vi "FSK_SEND_TEST.vi"() -> ()   [LabVIEW 2015]
doc: "Continuously generates a communication signal that starts immediately. The device is not synchronized to external Reference Clocks or time bases."
uses:
  <vilib>/Utility/error.llb/DialogType.ctl
  <instrlib>/niUSRP/niUSRP Write Tx Data (CDB).vi
panel:
  out "数据源长度":dbl=1000.0
  in  "码元速率":dbl=10000.0
  in  "信号长度":dbl=50000.0
  out "实际发射帧数":dbl=50.0 format="%#_6f"
  in  "设定发射帧数":dbl=50.0
  in  "数据源文件":path=path "C:/Users/admin/Desktop/USRP0902/USRP/Fsk/SendBit.mat"
  out "波形图":dbl[](graph)
  out "实际发射增益":dbl=10.0 format="%#_6f"
  in  "设备IP":refnum<k15>="192.168.10.2"
  in  "天线选择":string="TX1"
  in  "stop":bool
  out "实际载波频率":dbl=1000000000.0 format="%#_6p"
  out "实际基带采样率":dbl=200000.0 format="%#_6p"
  in  "设定发射增益":dbl=10.0 format="%#_6f"
  in  "设定载波频率":dbl=1000000000.0 format="%#_6p"
  in  "设定基带采样率":dbl=200000.0 format="%#_6p"
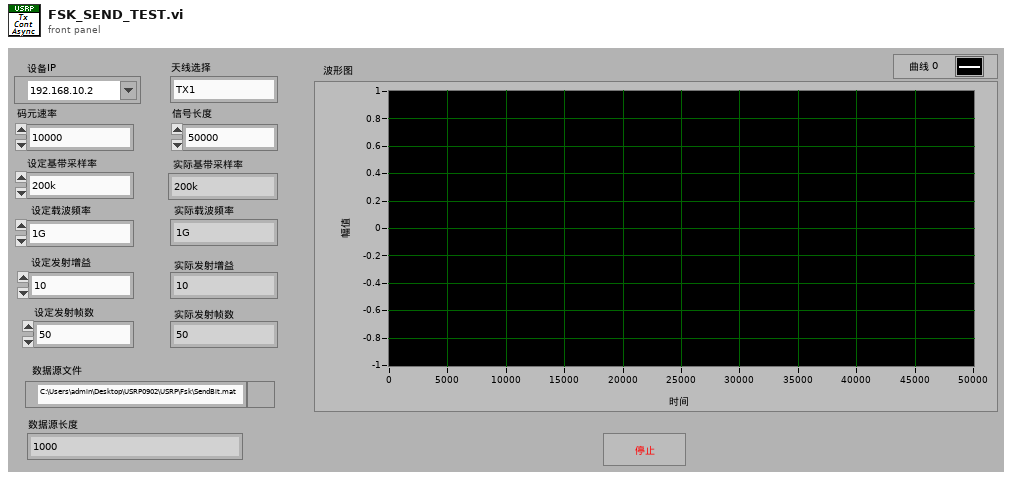
[diagram p1: front panel]
types:
  T1 = typedef "DialogType.ctl" = u16
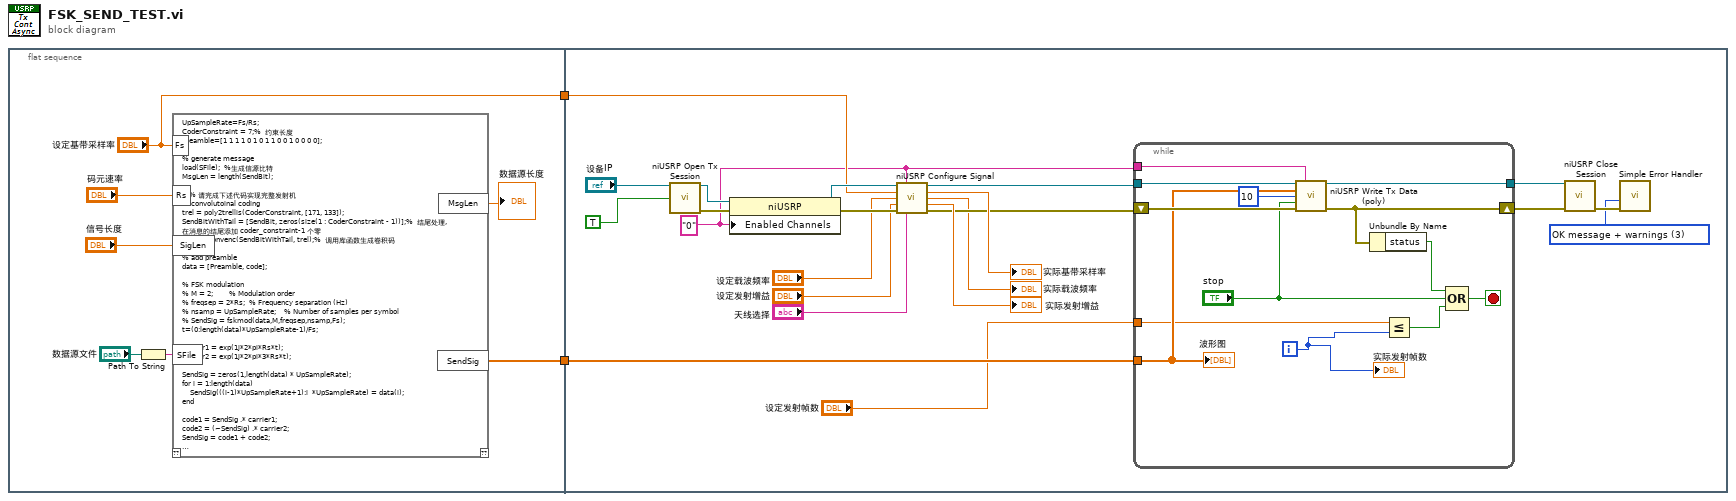
[diagram p0: block diagram]
diagram:
  n1 = flat-sequence {
    tunnel: ["设定基带采样率"] -> w2
    tunnel: [w6] -> w1
    tunnel: w2 -> [w13]
    tunnel: w1 -> [w12]
    frame #0 {
      n2 = Path To String(path="数据源文件") -> (string=w8:string)
      n3 = script code="UpSampleRate=Fs/Rs;\nCoderConstraint = 7;%  约束长度 \nPreamble=[1 1 1 1 0 1 0 1 1 0 0 1 0 0 0 0];\n\n% generate message\nload(SFile);  %生成信源比特\nMsgLen = length(SendBit);\n\n%% 请完成下述代码实现完整发射机\n% convolutoinal coding\ntrel = poly2trellis(CoderConstraint, [171, 133]);\nSendBitWithTail = [SendBit, zeros(size(1 : CoderConstraint - 1))];%  结尾处理, 在消息的结尾添加 coder_constraint-1 个零\ncode = convenc(SendBitWithTail, trel);%  调用库函数生成卷积码\n\n% add preamble \ndata = [Preamble, code];\n\n% FSK modulation\n% M = 2;        % Modulation order\n% freqsep = 2*Rs;  % Frequency separation (Hz)\n% nsamp = UpSampleRate;    % Number of samples per symbol\n% SendSig = fskmod(data,M,freqsep,nsamp,Fs);\nt=(0:length(data)*UpSampleRate-1)/Fs;\n\ncarrier1 = exp(1j*2*pi*Rs*t);\ncarrier2 = exp(1j*2*pi*3*Rs*t);\n\nSendSig = zeros(1,length(data) * UpSampleRate);\nfor i = 1:length(data)\n    SendSig(((i-1)*UpSampleRate+1):i  *UpSampleRate) = data(i);\nend\n\ncode1 = SendSig .* carrier1;\ncode2 = (~SendSig) .* carrier2;\nSendSig = code1 + code2;\n\n% 确保信号长度是SigLen\nif length(SendSig)>SigLen\n    SendSig = SendSig(1:SigLen);\nelseif length(SendSig)<SigLen\n    SendSig = [SendSig zeros(1,SigLen-length(SendSig))];\nend\nfigure;plot(SendBit);title('SendBit：数据源比特');\nfigure;plot(phasez(SendSig));title('phase(SendSig)：FSK发送信号相位');"("Fs"="设定基带采样率", "SFile"=w8, "Rs"="码元速率", "SigLen"="信号长度") -> ("SendSig"=w6:cdb[], "MsgLen"=→"数据源长度":dbl)  [unwired: 1 in, 1 out]
    }
    frame #1 {
      w11 = "0"
      w30 = T1 3 items=["no dialog", "OK message", "continue or stop message", "OK message + warnings", "continue/stop + warnings"] ("type of dialog (OK msg:1)")
      n4 = call <instrlib>:"niUSRP Open Tx Session.vi"("device names"="设备IP", "reset"=TRUE) -> ("session handle out"=w26:refnum<k15>, "error out"=w25:errorcluster)  [unwired: 12 in]
      n5 = property class="niUSRP"(reference=w26, error in=w25, "Enabled Channels"=w11) -> (reference out=w27:refnum<k15>, error out=w28:errorcluster)
      n6 = call <instrlib>:"niUSRP Configure Signal.vi"("session handle"=w27, "channel list"=w11, "IQ rate"=w13, "carrier frequency"="设定载波频率", "gain"="设定发射增益", "error in (no error)"=w28, "active antenna"="天线选择") -> ("session handle out"=w16:refnum<k15>, "coerced IQ rate"=→"实际基带采样率":dbl, "coerced carrier frequency"=→"实际载波频率":dbl, "coerced gain"=→"实际发射增益":dbl, "error out"=w17:errorcluster)  [unwired: 4 in]
      n7 = while {
        tunnel: w16 -> [w43]
        tunnel: [w41] -> w18
        shift-right: [w40] -> w19
        shift-left: w17 -> [w42]
        tunnel: w11 -> [w38]
        tunnel: w12 -> [w37]
        tunnel: "设定发射帧数" -> [w33]
        i -> [w32]
        stop <- w44 stop-if-true
        n8 = call-poly <instrlib>:"niUSRP Write Tx Data (poly).vi"("session handle"=w43, "channel list"=w38, "data"=w37, "timeout"=10, "end of data?"="stop", "error in (no error)"=w42) -> ("session handle out"=w41:refnum<k15>, "error out"=w40:errorcluster)  [unwired: 8 in]
        n9 = Unbundle By Name(w40) -> ("status"=w39:bool)
        n10 = Less Or Equal?(x=w33, y=w32) -> (x <= y?=w35:bool)
        n11 = Compound Arithmetic op=OR(w39, "stop", w35) -> (w44:bool)
        "波形图" <- w37
        "实际发射帧数" <- w32
      }
      n12 = call <instrlib>:"niUSRP Close Session.vi"("session handle"=w18, "error in (no error)"=w19) -> ("error out"=w31:errorcluster)  [unwired: 13 in]
      n13 = call <vilib>:"Simple Error Handler.vi"("type of dialog (OK msg:1)"=w30, "error in (no error)"=w31) -> ()  [unwired: 3 in, 5 out]
    }
  }
